vi "CreateDefaultDeviceNames.vi"(11 "DUT Count":i32) -> (3 "Default Device Names":string[](array[string]))   [LabVIEW 2013]
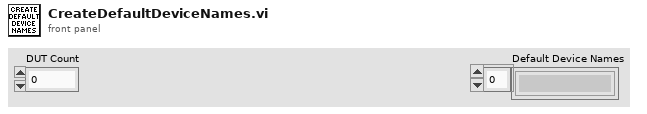
[diagram p1: front panel]
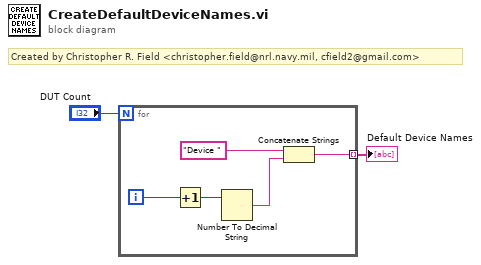
[diagram p0: block diagram]
diagram:
  # "Created by Christopher R. Field <christopher.field@nrl.navy.mil, cfield2@gmail.com>"
  n1 = for {
    N: "DUT Count" -> [_]
    tunnel: [w3] -> w1 mode=indexing
    i -> [w7]
    n2 = Increment(x=w7) -> (x+1=w6:i32)
    n3 = Number To Decimal String(number=w6) -> (decimal integer string=w4:string)  [unwired: 1 in]
    n4 = Concatenate Strings("Device ", w4) -> (w3:string)
  }
  "Default Device Names" <- w1
